vi "parse-xml_expSpec.vi"(6 "expSpecification XPath":cluster{"parameter":string, "datatype":string}[](array[cluster]), 8 "error in (no error)":errorcluster, 11 "expSpecification XML-String":string) -> (0 "error out":errorcluster, 3 "Input Array":variant[](array[variant]))   [LabVIEW 2013]
uses:
  <vilib>/xml/NI_XML.lvlib
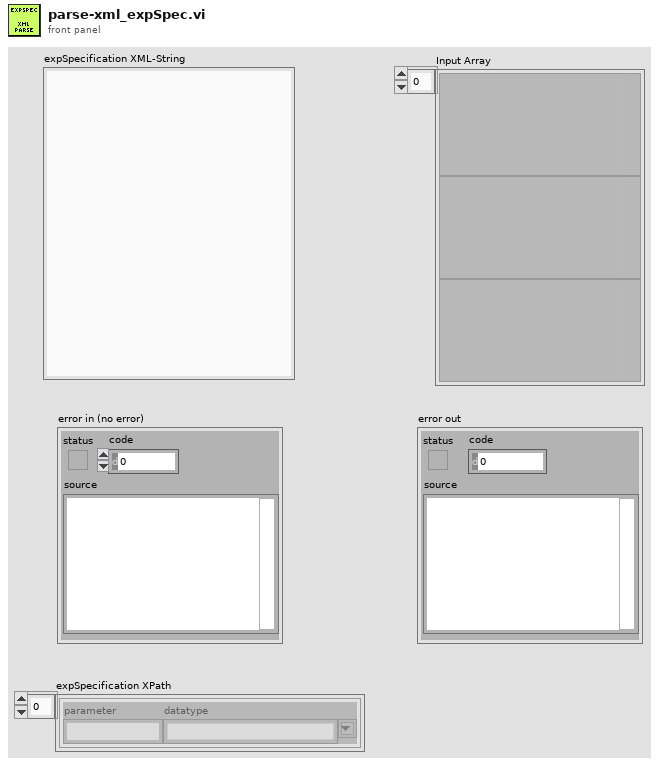
[diagram p1: front panel]
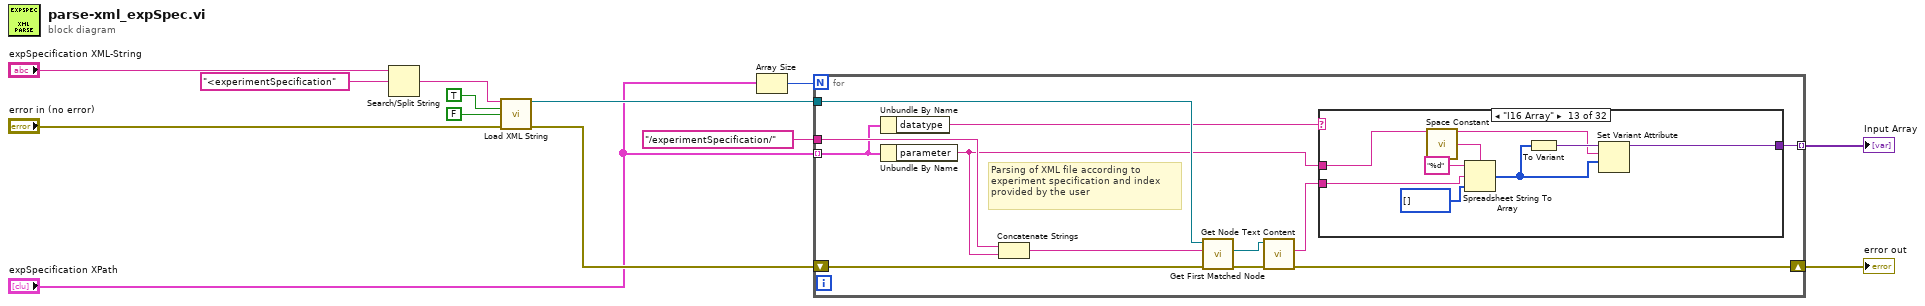
[diagram p0: block diagram]
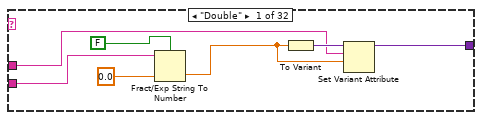
[diagram p2: hidden frame]
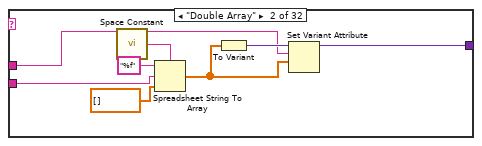
[diagram p3: hidden frame]
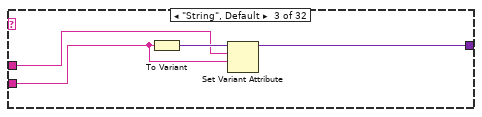
[diagram p4: hidden frame]
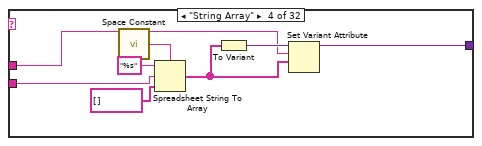
[diagram p5: hidden frame]
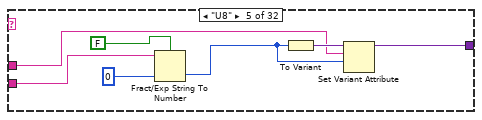
[diagram p6: hidden frame]
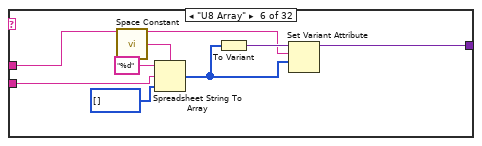
[diagram p7: hidden frame]
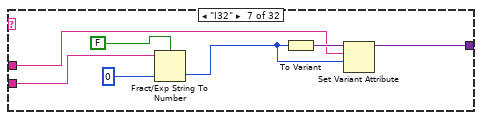
[diagram p8: hidden frame]
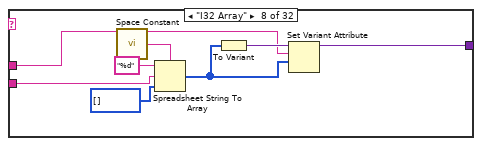
[diagram p9: hidden frame]
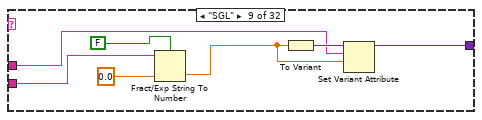
[diagram p10: hidden frame]
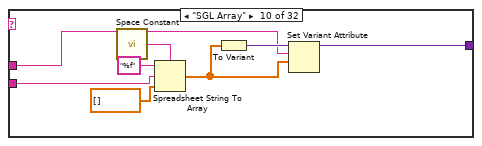
[diagram p11: hidden frame]
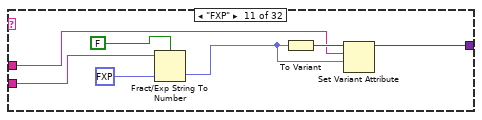
[diagram p12: hidden frame]
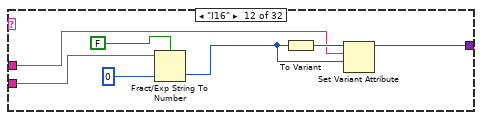
[diagram p13: hidden frame]
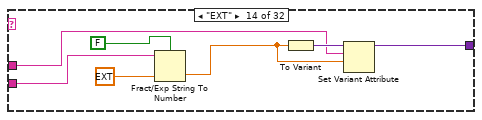
[diagram p14: hidden frame]
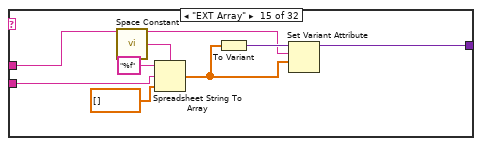
[diagram p15: hidden frame]
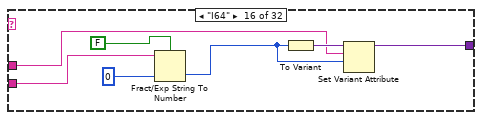
[diagram p16: hidden frame]
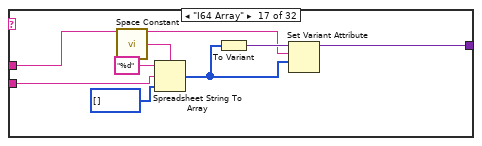
[diagram p17: hidden frame]
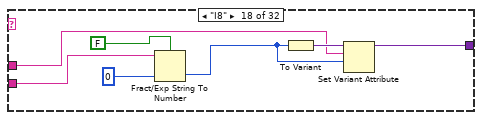
[diagram p18: hidden frame]
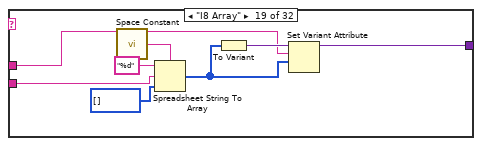
[diagram p19: hidden frame]
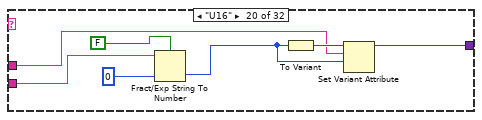
[diagram p20: hidden frame]
diagram:
  n1 = Search/Split String(string="expSpecification XML-String", search string/char (-)="<experimentSpecification") -> (match + rest of string=w9:string)  [unwired: 1 in, 2 out]
  n2 = call <vilib>:"Load XML String.vi"("XML string"=w9, "process namespaces (False)"=TRUE, "process schema (False)"=FALSE, "error in (no error)"="error in (no error)") -> ("DOM document out"=w11:refnum<k20>, "error out"=w7:errorcluster)  [unwired: 10 out]
  n3 = Array Size(array="expSpecification XPath") -> (size(s)=w8:i32)
  n4 = for {
    N: w8 -> [_]
    tunnel: w11 -> [w25]
    tunnel: "/experimentSpecification/" -> [w23]
    tunnel: "expSpecification XPath" -> [w21] mode=indexing
    tunnel: [w19] -> w2 mode=indexing
    shift-right: [w14] -> w3
    shift-left: w7 -> [w20]
    # "Parsing of XML file according to experiment specification and index provided by the user"
    n5 = Unbundle By Name(w21) -> ("datatype"=w18:string)
    n6 = Unbundle By Name(w21) -> ("parameter"=w16:string)
    n7 = Concatenate Strings(w23, w16) -> (w22:string)
    n8 = call <vilib>:"Get First Matched Node.vi"("error in (no error)"=w20, "XPath expression"=w22, "node in"=w25) -> ("error out"=w15:errorcluster, "node result"=w24:refnum<k20>)  [unwired: 6 in, 1 out]
    n9 = call <vilib>:"Get Node Text Content.vi"("error in (no error)"=w15, "node in"=w24) -> ("error out"=w14:errorcluster, "node text"=w17:string)  [unwired: 7 in, 1 out]
    n10 = case shown="\"I16 Array\"" w18 {
      tunnel: w16 -> [w26 w34 w41 w45 w53 w60 w68 w76 w83 w91 w98 w105 w112 w120 w128 w135 w142 w150 w157 w165 w172 w180 w187 w195 w202 w210 w218 w226 w233 w240 w248 w255]
      tunnel: w17 -> [w27 w33 w42 w46 w54 w61 w69 w75 w84 w90 w99 w106 w113 w121 w127 w136 w143 w151 w158 w166 w173 w181 w188 w196 w203 w211 w217 w225 w232 w241 w247 w256]
      tunnel: [w29 w36 w43 w49 w56 w64 w71 w79 w86 w93 w101 w108 w116 w123 w130 w138 w146 w153 w161 w168 w176 w183 w191 w198 w206 w213 w220 w228 w235 w243 w250 w258] -> w19
      frame "Double" {
        n11 = Fract/Exp String To Number(use system decimal point (T)=FALSE, string=w27, default (0 dbl)=0.0) -> (number=w28:dbl)  [unwired: 1 in, 1 out]
        n12 = To Variant(anything=w28) -> (Variant=w30:variant)
        n13 = Set Variant Attribute(Variant=w30, name=w26, value=w28) -> (Variant out=w29:variant)  [unwired: 1 in, 2 out]
      }
      frame "Double Array" {
        n14 = call <vilib>:"Space Constant.vi"() -> ("String"=w38:string)
        n15 = Spreadsheet String To Array(delimiter (Tab)=w38, format string="%f", spreadsheet string=w33, array type (2D Dbl)=dbl[] [] ("Array")) -> (array=w35:dbl[])
        n16 = To Variant(anything=w35) -> (Variant=w37:variant)
        n17 = Set Variant Attribute(Variant=w37, name=w34, value=w35) -> (Variant out=w36:variant)  [unwired: 1 in, 2 out]
      }
      frame "String", Default {
        n18 = To Variant(anything=w42) -> (Variant=w44:variant)
        n19 = Set Variant Attribute(Variant=w44, name=w41, value=w42) -> (Variant out=w43:variant)  [unwired: 1 in, 2 out]
      }
      frame "String Array" {
        n20 = call <vilib>:"Space Constant.vi"() -> ("String"=w51:string)
        n21 = Spreadsheet String To Array(delimiter (Tab)=w51, format string="%s", spreadsheet string=w46, array type (2D Dbl)=string[] [] ("Array")) -> (array=w48:string[])
        n22 = To Variant(anything=w48) -> (Variant=w50:variant)
        n23 = Set Variant Attribute(Variant=w50, name=w45, value=w48) -> (Variant out=w49:variant)  [unwired: 1 in, 2 out]
      }
      frame "U8" {
        n24 = Fract/Exp String To Number(use system decimal point (T)=FALSE, string=w54, default (0 dbl)=u8 0) -> (number=w55:u8)  [unwired: 1 in, 1 out]
        n25 = To Variant(anything=w55) -> (Variant=w57:variant)
        n26 = Set Variant Attribute(Variant=w57, name=w53, value=w55) -> (Variant out=w56:variant)  [unwired: 1 in, 2 out]
      }
      frame "U8 Array" {
        n27 = call <vilib>:"Space Constant.vi"() -> ("String"=w66:string)
        n28 = Spreadsheet String To Array(delimiter (Tab)=w66, format string="%d", spreadsheet string=w61, array type (2D Dbl)=u8[] [] ("Array")) -> (array=w62:u8[])
        n29 = To Variant(anything=w62) -> (Variant=w65:variant)
        n30 = Set Variant Attribute(Variant=w65, name=w60, value=w62) -> (Variant out=w64:variant)  [unwired: 1 in, 2 out]
      }
      frame "I32" {
        n31 = Fract/Exp String To Number(use system decimal point (T)=FALSE, string=w69, default (0 dbl)=0) -> (number=w70:i32)  [unwired: 1 in, 1 out]
        n32 = To Variant(anything=w70) -> (Variant=w72:variant)
        n33 = Set Variant Attribute(Variant=w72, name=w68, value=w70) -> (Variant out=w71:variant)  [unwired: 1 in, 2 out]
      }
      frame "I32 Array" {
        n34 = call <vilib>:"Space Constant.vi"() -> ("String"=w81:string)
        n35 = Spreadsheet String To Array(delimiter (Tab)=w81, format string="%d", spreadsheet string=w75, array type (2D Dbl)=i32[] [] ("Array")) -> (array=w77:i32[])
        n36 = To Variant(anything=w77) -> (Variant=w80:variant)
        n37 = Set Variant Attribute(Variant=w80, name=w76, value=w77) -> (Variant out=w79:variant)  [unwired: 1 in, 2 out]
      }
      frame "SGL" {
        n38 = Fract/Exp String To Number(use system decimal point (T)=FALSE, string=w84, default (0 dbl)=sgl 0.0) -> (number=w85:sgl)  [unwired: 1 in, 1 out]
        n39 = To Variant(anything=w85) -> (Variant=w87:variant)
        n40 = Set Variant Attribute(Variant=w87, name=w83, value=w85) -> (Variant out=w86:variant)  [unwired: 1 in, 2 out]
      }
      frame "SGL Array" {
        n41 = call <vilib>:"Space Constant.vi"() -> ("String"=w95:string)
        n42 = Spreadsheet String To Array(delimiter (Tab)=w95, format string="%f", spreadsheet string=w90, array type (2D Dbl)=sgl[] [] ("Array")) -> (array=w92:sgl[])
        n43 = To Variant(anything=w92) -> (Variant=w94:variant)
        n44 = Set Variant Attribute(Variant=w94, name=w91, value=w92) -> (Variant out=w93:variant)  [unwired: 1 in, 2 out]
      }
      frame "FXP" {
        n45 = Fract/Exp String To Number(use system decimal point (T)=FALSE, string=w99, default (0 dbl)=fxp<+,1,1> 0.0) -> (number=w100:fxp<+,1,1>)  [unwired: 1 in, 1 out]
        n46 = To Variant(anything=w100) -> (Variant=w102:variant)
        n47 = Set Variant Attribute(Variant=w102, name=w98, value=w100) -> (Variant out=w101:variant)  [unwired: 1 in, 2 out]
      }
      frame "I16" {
        n48 = Fract/Exp String To Number(use system decimal point (T)=FALSE, string=w106, default (0 dbl)=i16 0 ("I16")) -> (number=w109:i16)  [unwired: 1 in, 1 out]
        n49 = To Variant(anything=w109) -> (Variant=w110:variant)
        n50 = Set Variant Attribute(Variant=w110, name=w105, value=w109) -> (Variant out=w108:variant)  [unwired: 1 in, 2 out]
      }
      frame "I16 Array" {
        n51 = call <vilib>:"Space Constant.vi"() -> ("String"=w118:string)
        n52 = Spreadsheet String To Array(delimiter (Tab)=w118, format string="%d", spreadsheet string=w113, array type (2D Dbl)=i16[] [] ("Array")) -> (array=w114:i16[])
        n53 = To Variant(anything=w114) -> (Variant=w117:variant)
        n54 = Set Variant Attribute(Variant=w117, name=w112, value=w114) -> (Variant out=w116:variant)  [unwired: 1 in, 2 out]
      }
      frame "EXT" {
        n55 = Fract/Exp String To Number(use system decimal point (T)=FALSE, string=w121, default (0 dbl)=ext 0.0) -> (number=w122:ext)  [unwired: 1 in, 1 out]
        n56 = To Variant(anything=w122) -> (Variant=w124:variant)
        n57 = Set Variant Attribute(Variant=w124, name=w120, value=w122) -> (Variant out=w123:variant)  [unwired: 1 in, 2 out]
      }
      frame "EXT Array" {
        n58 = call <vilib>:"Space Constant.vi"() -> ("String"=w132:string)
        n59 = Spreadsheet String To Array(delimiter (Tab)=w132, format string="%f", spreadsheet string=w127, array type (2D Dbl)=ext[] [] ("Array")) -> (array=w129:ext[])
        n60 = To Variant(anything=w129) -> (Variant=w131:variant)
        n61 = Set Variant Attribute(Variant=w131, name=w128, value=w129) -> (Variant out=w130:variant)  [unwired: 1 in, 2 out]
      }
      frame "I64" {
        n62 = Fract/Exp String To Number(use system decimal point (T)=FALSE, string=w136, default (0 dbl)=i64 0) -> (number=w137:i64)  [unwired: 1 in, 1 out]
        n63 = To Variant(anything=w137) -> (Variant=w139:variant)
        n64 = Set Variant Attribute(Variant=w139, name=w135, value=w137) -> (Variant out=w138:variant)  [unwired: 1 in, 2 out]
      }
      frame "I64 Array" {
        n65 = call <vilib>:"Space Constant.vi"() -> ("String"=w148:string)
        n66 = Spreadsheet String To Array(delimiter (Tab)=w148, format string="%d", spreadsheet string=w143, array type (2D Dbl)=i64[] [] ("Array")) -> (array=w144:i64[])
        n67 = To Variant(anything=w144) -> (Variant=w147:variant)
        n68 = Set Variant Attribute(Variant=w147, name=w142, value=w144) -> (Variant out=w146:variant)  [unwired: 1 in, 2 out]
      }
      frame "I8" {
        n69 = Fract/Exp String To Number(use system decimal point (T)=FALSE, string=w151, default (0 dbl)=i8 0) -> (number=w152:i8)  [unwired: 1 in, 1 out]
        n70 = To Variant(anything=w152) -> (Variant=w154:variant)
        n71 = Set Variant Attribute(Variant=w154, name=w150, value=w152) -> (Variant out=w153:variant)  [unwired: 1 in, 2 out]
      }
      frame "I8 Array" {
        n72 = call <vilib>:"Space Constant.vi"() -> ("String"=w163:string)
        n73 = Spreadsheet String To Array(delimiter (Tab)=w163, format string="%d", spreadsheet string=w158, array type (2D Dbl)=i8[] [] ("Array")) -> (array=w159:i8[])
        n74 = To Variant(anything=w159) -> (Variant=w162:variant)
        n75 = Set Variant Attribute(Variant=w162, name=w157, value=w159) -> (Variant out=w161:variant)  [unwired: 1 in, 2 out]
      }
      frame "U16" {
        n76 = Fract/Exp String To Number(use system decimal point (T)=FALSE, string=w166, default (0 dbl)=u16 0) -> (number=w167:u16)  [unwired: 1 in, 1 out]
        n77 = To Variant(anything=w167) -> (Variant=w169:variant)
        n78 = Set Variant Attribute(Variant=w169, name=w165, value=w167) -> (Variant out=w168:variant)  [unwired: 1 in, 2 out]
      }
      frame "U16 Array" {
        n79 = call <vilib>:"Space Constant.vi"() -> ("String"=w178:string)
        n80 = Spreadsheet String To Array(delimiter (Tab)=w178, format string="%d", spreadsheet string=w173, array type (2D Dbl)=u16[] [] ("Array")) -> (array=w174:u16[])
        n81 = To Variant(anything=w174) -> (Variant=w177:variant)
        n82 = Set Variant Attribute(Variant=w177, name=w172, value=w174) -> (Variant out=w176:variant)  [unwired: 1 in, 2 out]
      }
      frame "U32" {
        n83 = Fract/Exp String To Number(use system decimal point (T)=FALSE, string=w181, default (0 dbl)=u32 0) -> (number=w182:u32)  [unwired: 1 in, 1 out]
        n84 = To Variant(anything=w182) -> (Variant=w184:variant)
        n85 = Set Variant Attribute(Variant=w184, name=w180, value=w182) -> (Variant out=w183:variant)  [unwired: 1 in, 2 out]
      }
      frame "U32 Array" {
        n86 = call <vilib>:"Space Constant.vi"() -> ("String"=w193:string)
        n87 = Spreadsheet String To Array(delimiter (Tab)=w193, format string="%d", spreadsheet string=w188, array type (2D Dbl)=u32[] [] ("Array")) -> (array=w189:u32[])
        n88 = To Variant(anything=w189) -> (Variant=w192:variant)
        n89 = Set Variant Attribute(Variant=w192, name=w187, value=w189) -> (Variant out=w191:variant)  [unwired: 1 in, 2 out]
      }
      frame "U64" {
        n90 = Fract/Exp String To Number(use system decimal point (T)=FALSE, string=w196, default (0 dbl)=u64 0) -> (number=w197:u64)  [unwired: 1 in, 1 out]
        n91 = To Variant(anything=w197) -> (Variant=w199:variant)
        n92 = Set Variant Attribute(Variant=w199, name=w195, value=w197) -> (Variant out=w198:variant)  [unwired: 1 in, 2 out]
      }
      frame "U64 Array" {
        n93 = call <vilib>:"Space Constant.vi"() -> ("String"=w208:string)
        n94 = Spreadsheet String To Array(delimiter (Tab)=w208, format string="%d", spreadsheet string=w203, array type (2D Dbl)=u64[] [] ("Array")) -> (array=w204:u64[])
        n95 = To Variant(anything=w204) -> (Variant=w207:variant)
        n96 = Set Variant Attribute(Variant=w207, name=w202, value=w204) -> (Variant out=w206:variant)  [unwired: 1 in, 2 out]
      }
      frame "CXT" {
        n97 = Scan From String(format string="%f", input string=w211, default 1=cxt 0.0+0.0i ("number 3")) -> (output 1=w212:cxt)  [unwired: 2 in, 3 out]
        n98 = To Variant(anything=w212) -> (Variant=w214:variant)
        n99 = Set Variant Attribute(Variant=w214, name=w210, value=w212) -> (Variant out=w213:variant)  [unwired: 1 in, 2 out]
      }
      frame "CXT Array" {
        n100 = call <vilib>:"Space Constant.vi"() -> ("String"=w222:string)
        n101 = Spreadsheet String To Array(delimiter (Tab)=w222, format string="%f", spreadsheet string=w217, array type (2D Dbl)=cxt[] [] ("Array")) -> (array=w219:cxt[])
        n102 = To Variant(anything=w219) -> (Variant=w221:variant)
        n103 = Set Variant Attribute(Variant=w221, name=w218, value=w219) -> (Variant out=w220:variant)  [unwired: 1 in, 2 out]
      }
      frame "CDB" {
        n104 = Scan From String(format string="%f", input string=w225, default 1=cdb 0.0+0.0i ("number 3")) -> (output 1=w227:cdb)  [unwired: 2 in, 3 out]
        n105 = To Variant(anything=w227) -> (Variant=w229:variant)
        n106 = Set Variant Attribute(Variant=w229, name=w226, value=w227) -> (Variant out=w228:variant)  [unwired: 1 in, 2 out]
      }
      frame "CDB Array" {
        n107 = call <vilib>:"Space Constant.vi"() -> ("String"=w237:string)
        n108 = Spreadsheet String To Array(delimiter (Tab)=w237, format string="%f", spreadsheet string=w232, array type (2D Dbl)=cdb[] [] ("Array")) -> (array=w234:cdb[])
        n109 = To Variant(anything=w234) -> (Variant=w236:variant)
        n110 = Set Variant Attribute(Variant=w236, name=w233, value=w234) -> (Variant out=w235:variant)  [unwired: 1 in, 2 out]
      }
      frame "CSG" {
        n111 = Scan From String(format string="%f", input string=w241, default 1=csg 0.0+0.0i ("number 3")) -> (output 1=w242:csg)  [unwired: 2 in, 3 out]
        n112 = To Variant(anything=w242) -> (Variant=w244:variant)
        n113 = Set Variant Attribute(Variant=w244, name=w240, value=w242) -> (Variant out=w243:variant)  [unwired: 1 in, 2 out]
      }
      frame "CSG Array" {
        n114 = call <vilib>:"Space Constant.vi"() -> ("String"=w252:string)
        n115 = Spreadsheet String To Array(delimiter (Tab)=w252, format string="%f", spreadsheet string=w247, array type (2D Dbl)=csg[] [] ("Array")) -> (array=w249:csg[])
        n116 = To Variant(anything=w249) -> (Variant=w251:variant)
        n117 = Set Variant Attribute(Variant=w251, name=w248, value=w249) -> (Variant out=w250:variant)  [unwired: 1 in, 2 out]
      }
      frame "Boolean" {
        n118 = case shown="\"False\", Default" w256 {
          tunnel: [FALSE TRUE TRUE FALSE TRUE FALSE TRUE FALSE] -> w257
          frame "False", Default {
          }
          frame "True" {
          }
          frame "TRUE" {
          }
          frame "FALSE" {
          }
          frame "1" {
          }
          frame "0" {
          }
          frame "true" {
          }
          frame "false" {
          }
        }
        n119 = To Variant(anything=w257) -> (Variant=w259:variant)
        n120 = Set Variant Attribute(Variant=w259, name=w255, value=w257) -> (Variant out=w258:variant)  [unwired: 1 in, 2 out]
      }
    }
  }
  "error out" <- w3
  "Input Array" <- w2
